vi "Contour.vi"(8 "Index":i32, 10 "VertexArray":T1[](array[typedef]), 11 "DocIn":refnum<k20>) -> (2 "Contour":refnum<k20>, 3 "DocOut":refnum<k20>)   [LabVIEW 2014]
uses:
  TypeDefs/Point2DwSlope.ctl
  <resource>/objmgr/DOMUserDefRef.rc
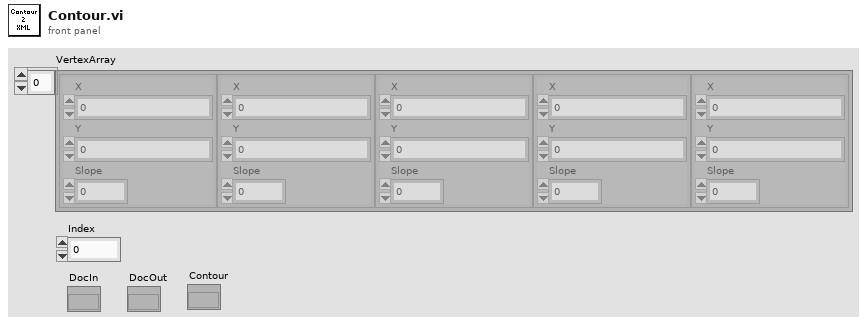
[diagram p1: front panel]
types:
  T1 = typedef "Point2DwSlope.ctl" = cluster{"X":sgl, "Y":sgl, "Slope":dbl}
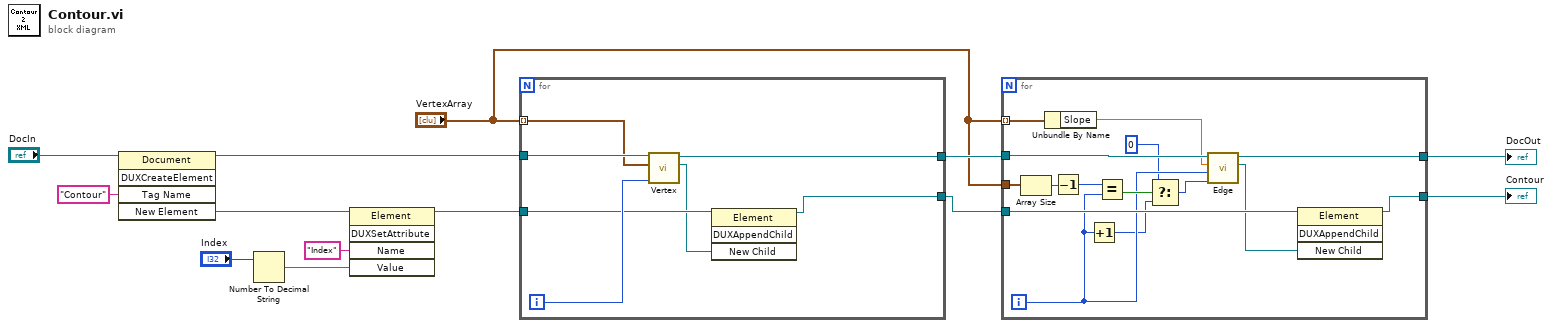
[diagram p0: block diagram]
diagram:
  n1 = invoke class="Document" method="DUXCreateElement"(reference="DocIn", "Tag Name"="Contour") -> (reference out=w12:refnum<k20>, "New Element"=w8:refnum<k20>)  [unwired: 3 in, 3 out]
  n2 = Number To Decimal String(number="Index") -> (decimal integer string=w10:string)  [unwired: 1 in]
  n3 = invoke class="Element" method="DUXSetAttribute"(reference=w8, "Name"="Index", "Value"=w10) -> (reference out=w7:refnum<k20>)  [unwired: 2 in, 4 out]
  n4 = for {
    tunnel: "VertexArray" -> [w19] mode=indexing
    tunnel: w12 -> [w20]
    tunnel: [w17] -> w5
    tunnel: w7 -> [w16]
    tunnel: [w14] -> w4
    i -> [w18]
    n5 = call "Vertex.vi"("Index"=w18, "Point2D"=w19, "DocIn"=w20) -> ("Vertex"=w15:refnum<k20>, "DocOut"=w17:refnum<k20>)  [unwired: 7 in]
    n6 = invoke class="Element" method="DUXAppendChild"(reference=w16, "New Child"=w15) -> (reference out=w14:refnum<k20>)  [unwired: 2 in, 3 out]
  }
  n7 = for {
    tunnel: "VertexArray" -> [w33] mode=indexing
    tunnel: w5 -> [w29]
    tunnel: w4 -> [w35]
    tunnel: [w34] -> w6
    tunnel: "VertexArray" -> [w32]
    tunnel: [w21] -> w2
    i -> [w26]
    n8 = Array Size(array=w32) -> (size(s)=w31:i32)
    n9 = Unbundle By Name(w33) -> ("Slope"=w23:dbl)
    n10 = Decrement(x=w31) -> (x-1=w30:i32)
    n11 = Increment(x=w26) -> (x+1=w25:i32)
    n12 = Equal?(x=w30, y=w26) -> (x = y?=w27:bool)
    n13 = Select(t=0, s=w27, f=w25) -> (s? t:f=w28:i32)
    n14 = call "Edge.vi"("Index2"=w28, "Index1"=w26, "Slope"=w23, "DocIn"=w29) -> ("Edge"=w22:refnum<k20>, "DocOut"=w21:refnum<k20>)  [unwired: 6 in]
    n15 = invoke class="Element" method="DUXAppendChild"(reference=w35, "New Child"=w22) -> (reference out=w34:refnum<k20>)  [unwired: 2 in, 3 out]
  }
  "DocOut" <- w2
  "Contour" <- w6
